vi "2P_AdapUprite_Linlin.vi"() -> ()   [LabVIEW 2015] (continued)
                                n1300 = local read "avpp"() -> (w4003:i32)
                                n1301 = call "tt_timeandsamples.vi"("bin"=w3997, "refreshtime"=w3991, "srateAODOtt"=w3994, "tot#ofsamples"=w3999) -> ("refreshrate"=w3995:dbl, "refreshbuffer"=w3996:i32, "timetracecycles"=w4001:i32)  [unwired: 5 in]
                                n1302 = local read "bin"() -> (w3998:dbl)
                                n1303 = call "2pparameters.vi"("command"="get") -> ("params out"=w4010:T12)  [unwired: 1 in]
                                n1304 = Bundle By Name(cluster=w4010, "Drawing Mode"=w3971, "measpoints"=w3999, "tt_cycles"=w4001, "refreshbuffer"=w3996, "refreshrate"=w3995, "Vx-ref"=w4002, "Vy-ref"=w4004, "srate"=w3993, "finite"=w4006, "cont"=w4005, "wavdet"=w4007, "avpp"=w4003, "srateAODO"=w4000, "bufferAI"=w3996, "bin"=w3998, "Angle Img"=w3978, "Vxminref"=w3977, "Vxmaxref"=w3976, "Vyminref"=w3975, "Vymaxref"=w3974, "Xpixels Img"=w3973, "Ypixels Img"=w3972, "Pel"=w3970, "Vz-reset"=0.0, "AIoverride"=w3968) -> (w4008:T12)
                                n1305 = Reciprocal(x=w3995) -> (1/x=w3992:dbl)
                                n1306 = local write "refreshtime"(w3992) -> ()
                                n1307 = call "2pparameters.vi"("Params in"=w4008, "command"="set") -> ()  [unwired: 1 out]
                                n1308 = local read "Voltage Clamp"() -> (w3985:bool)
                                n1309 = local read "Current Clamp"() -> (w3986:bool)
                                n1310 = local read "Vholding (mV)"() -> (w3980:sgl)
                                n1311 = local read "CC_ICgain"() -> (w3984:dbl)
                                n1312 = local read "OCgain"() -> (w3981:sgl)
                                n1313 = local read "holdon"() -> (w3979:bool)
                                n1314 = call "patchparameters.vi"("command"="get") -> ("Params out"=w3988:T16)  [unwired: 1 in]
                                n1315 = Bundle By Name(cluster=w3988, "VC"=w3985, "CC"=w3986, "CC_icg (pA/mv)"=w3984, "VC_icg (mV/mV)"=10.0, "OCG (mV/pA)"=w3981, "OVG (mV/mV)"=0.1, "Vhold (mV)"=w3980, "holdon"=w3979) -> (w3987:T16)
                                n1316 = call "patchparameters.vi"("Params in"=w3987, "command"="set") -> ()  [unwired: 1 out]
                              }
                              frame #4 {
                                # "calculating the waveform from the drawing"
                                n1317 = case shown="\"freeform contour\"" w4012 {
                                frame "Point" {
                                n1318 = call "2pparameters.vi"("command"="get") -> ("params out"=w4028:T12)  [unwired: 1 in]
                                n1319 = Unbundle By Name(w4028) -> ("Pel"=w4017:sgl, "Vx-min Img"=w4030:dbl, "VX-max Img"=w4029:dbl, "Vy-min Img"=w4032:dbl, "Vy-max Img"=w4031:dbl, "Angle Img"=w4033:dbl, "Vx-ref"=w4026:dbl, "Vy-ref"=w4025:dbl)
                                n1320 = script code="Xic=(ximax+ximin)./2;\nYic=(yimax+yimin)./2;\nx=x-Xic;\ny=y-Yic;\nxout=x.*cos(pi/180.*phi)+y.*sin(pi./180.*phi)+Xic;\nyout=-x.*sin(pi./180.*phi)+y.*cos(pi./180.*phi)+Yic;"("ximax"=w4029, "ximin"=w4030, "yimax"=w4031, "yimin"=w4032, "phi"=w4033, "x"=w4026, "y"=w4025) -> ("xout"=w4019:dbl, "yout"=w4018:dbl)  [unwired: 1 in, 1 out]
                                n1321 = call "2pparameters.vi"("command"="get") -> ("params out"=w4021:T12)  [unwired: 1 in]
                                n1322 = Bundle By Name(cluster=w4021, "P"=0.0) -> (w4024:T12)
                                n1323 = Initialize Array(w4018, w4017) -> (w4015:dbl[])
                                n1324 = Initialize Array(w4019, w4017) -> (w4014:dbl[])
                                n1325 = call "2pparameters.vi"("Params in"=w4024, "command"="set") -> ()  [unwired: 1 out]
                                n1326 = call "X-array-databuffer.vi"("array in"=w4014, "command"=enum16{"get", "set", "clear", "append"}."set") -> ()  [unwired: 2 in, 2 out]
                                n1327 = call "Y-array-databuffer.vi"("array in"=w4015, "command"=enum16{"get", "set", "clear", "append"}."set") -> ()  [unwired: 2 in, 2 out]
                                }
                                frame "Resonant Ellipse", Default {
                                n1328 = call "2pparameters.vi"("command"="get") -> ("params out"=w4048:T12)  [unwired: 1 in]
                                n1329 = Unbundle By Name(w4048) -> ("srateAODO"=w4049:sgl, "Angle Img"=w4050:dbl, "Angle draw"=w4051:dbl, "Vxmaxref"=w4052:dbl, "Vxminref"=w4053:dbl, "Xpixels Img"=w4054:i32, "Ypixels Img"=w4055:i32, "Vymaxref"=w4056:dbl, "Vyminref"=w4057:dbl, "Drawing Mode"=w4058:u16, "Pel"=w4059:sgl)
                                n1330 = Add(x=w4050, y=w4051) -> (x+y=w4034:dbl)
                                n1331 = call "ROI-databuffer.vi"("command"=enum16{"get", "set", "clear", "append"}."get") -> ("array out"=w4042:cluster{"x":sgl, "y":sgl}[])  [unwired: 4 in]
                                n1332 = call "ScanningWaveform_v4.vi"("Vy-min"=w4057, "Vy-max"=w4056, "yPixels/tPixels"=w4055, "xPixels/rPixels"=w4054, "Vx-min"=w4053, "Vx-max"=w4052, "Drawing Mode"=w4058, "Angle"=w4034, "AOrate"=w4049, "Points"=w4042, "points in ellipse"=w4059) -> ("numPixels"=w4035:dbl, "Y-WaveArray"=w4036:dbl[], "P"=w4041:dbl, "X-WaveArray"=w4037:dbl[])  [unwired: 5 in]
                                n1333 = call "Y-array-databuffer.vi"("array in"=w4036, "command"=enum16{"get", "set", "clear", "append"}."set") -> ()  [unwired: 2 in, 2 out]
                                n1334 = call "X-array-databuffer.vi"("array in"=w4037, "command"=enum16{"get", "set", "clear", "append"}."set") -> ()  [unwired: 2 in, 2 out]
                                n1335 = call "2pparameters.vi"("command"="get") -> ("params out"=w4046:T12)  [unwired: 1 in]
                                n1336 = Bundle By Name(cluster=w4046, "P"=w4041, "sAOxy"=w4035, "Pel"=w4035) -> (w4038:T12)
                                n1337 = call "2pparameters.vi"("Params in"=w4038, "command"="set") -> ()  [unwired: 1 out]
                                }
                                frame "freeform contour" {
                                n1338 = disable-structure shown="Enabled" {
                                frame Disabled {
                                # "Started writing this because old one was crashing....\nI think I found the source of the crash and was able to fix old one\n-Simon"
                                n1339 = call "2pparameters.vi"("command"="get") -> ("params out"=w4073:T12)  [unwired: 1 in]
                                n1340 = Unbundle By Name(w4073) -> ("Pel"=w4062:sgl)  [unwired: 10 out]
                                n1341 = call "ROI-databuffer.vi"("command"=enum16{"get", "set", "clear", "append"}."get") -> ("array out"=w4063:cluster{"x":sgl, "y":sgl}[])  [unwired: 4 in]
                                n1342 = call "Contour_ToVolts.vi"("N Contour Points"=w4062, "Array In"=w4063) -> ("Y Array Out"=w4060:dbl[], "X Array Out"=w4061:dbl[])  [unwired: 8 in]
                                n1343 = call "2pparameters.vi"("command"="get") -> ("params out"=w4071:T12)  [unwired: 1 in]
                                n1344 = Bundle By Name(cluster=w4071, "P"=0.0, "sAOxy"=w4062, "Pel"=w4062) -> (w4065:T12)
                                n1345 = call "Y-array-databuffer.vi"("array in"=w4060, "command"=enum16{"get", "set", "clear", "append"}."set") -> ()  [unwired: 2 in, 2 out]
                                n1346 = call "X-array-databuffer.vi"("array in"=w4061, "command"=enum16{"get", "set", "clear", "append"}."set") -> ()  [unwired: 2 in, 2 out]
                                n1347 = call "2pparameters.vi"("Params in"=w4065, "command"="set") -> ()  [unwired: 1 out]
                                }
                                frame Enabled {
                                n1348 = call "2pparameters.vi"("command"="get") -> ("params out"=w4088:T12)  [unwired: 1 in]
                                n1349 = Unbundle By Name(w4088) -> ("srateAODO"=w4089:sgl, "Angle Img"=w4090:dbl, "Angle draw"=w4091:dbl, "Vxmaxref"=w4092:dbl, "Vxminref"=w4093:dbl, "Xpixels Img"=w4094:i32, "Ypixels Img"=w4095:i32, "Vymaxref"=w4096:dbl, "Vyminref"=w4097:dbl, "Drawing Mode"=w4098:u16, "Pel"=w4099:sgl)
                                n1350 = Add(x=w4090, y=w4091) -> (x+y=w4074:dbl)
                                n1351 = call "ROI-databuffer.vi"("command"=enum16{"get", "set", "clear", "append"}."get") -> ("array out"=w4082:cluster{"x":sgl, "y":sgl}[])  [unwired: 4 in]
                                n1352 = call "ScanningWaveform_v4.vi"("Vy-min"=w4097, "Vy-max"=w4096, "yPixels/tPixels"=w4095, "xPixels/rPixels"=w4094, "Vx-min"=w4093, "Vx-max"=w4092, "Drawing Mode"=w4098, "Angle"=w4074, "AOrate"=w4089, "Points"=w4082, "points in ellipse"=w4099) -> ("numPixels"=w4075:dbl, "Y-WaveArray"=w4076:dbl[], "P"=w4081:dbl, "X-WaveArray"=w4077:dbl[])  [unwired: 5 in]
                                n1353 = call "Y-array-databuffer.vi"("array in"=w4076, "command"=enum16{"get", "set", "clear", "append"}."set") -> ()  [unwired: 2 in, 2 out]
                                n1354 = call "X-array-databuffer.vi"("array in"=w4077, "command"=enum16{"get", "set", "clear", "append"}."set") -> ()  [unwired: 2 in, 2 out]
                                n1355 = call "2pparameters.vi"("command"="get") -> ("params out"=w4086:T12)  [unwired: 1 in]
                                n1356 = Bundle By Name(cluster=w4086, "P"=w4081, "sAOxy"=w4075, "Pel"=w4075) -> (w4078:T12)
                                n1357 = call "2pparameters.vi"("Params in"=w4078, "command"="set") -> ()  [unwired: 1 out]
                                }
                                }
                                }
                                }
                              }
                              frame #5 {
                                # "set starting position"
                                n1358 = call "X-array-databuffer.vi"("command"=enum16{"get", "set", "clear", "append"}."get") -> ("array out"=w4102:dbl[])  [unwired: 3 in, 1 out]
                                n1359 = call "Y-array-databuffer.vi"("command"=enum16{"get", "set", "clear", "append"}."get") -> ("array out"=w4105:dbl[])  [unwired: 3 in, 1 out]
                                n1360 = Index Array(array=w4102, index=0) -> (element=w4101:dbl)
                                n1361 = Index Array(array=w4105, index=0) -> (element=w4100:dbl)
                                n1362 = call "setposition.vi"("Vy"=w4100, "Vx"=w4101) -> ()  [unwired: 1 in]
                              }
                              frame #6 {
                                # "rem2Ps"
                                # "A2Ps"
                                # "Al"
                                # "Rl"
                                # "Here it is writing the contour to a waveform that will be given to the AO (and also DO)"
                                n1363 = stacked-sequence {
                                seq-local: [w4126 _ _ _ _ _ _ _ _ _ _] -> [_ w4246 _ w4307 _ w4393 _ _ _ _ _]
                                seq-local: [w4127 _ _ _ _ _ _ _ _ _ _] -> [_ w4247 w4257 _ w4362 _ _ _ _ _ _]
                                seq-local: [_ _ w4256 _ _ _ _ _ _ _ _] -> [_ _ _ _ w4356 _ _ _ _ _ _]
                                seq-local: [_ _ _ w4306 _ _ _ _ _ _ _] -> [_ _ _ _ _ w4392 _ _ _ _ _]
                                seq-local: [w4123 _ _ _ _ _ _ _ _ _ _] -> [_ w4243 _ _ _ _ _ _ w4602 w4670 _]
                                seq-local: [w4122 _ _ _ _ _ _ _ _ _ _] -> [_ w4242 _ _ _ _ _ _ w4603 w4671 _]
                                seq-local: [w4129 _ _ _ _ _ _ _ _ _ _] -> [_ _ _ _ _ _ w4427 _ w4601 w4669 _]
                                seq-local: [w4125 _ _ _ _ _ _ _ _ _ _] -> [_ w4241 _ _ _ _ w4429 w4510 _ _ _]
                                seq-local: [w4124 _ _ _ _ _ _ _ _ _ _] -> [_ w4240 _ _ _ _ w4428 w4509 _ _ _]
                                seq-local: [w4128 _ _ _ _ _ _ _ _ _ _] -> [_ _ _ _ _ _ w4430 w4506 _ _ _]
                                tunnel: [_ _ w4255 _ _ _ _ _ _ _ _] -> w4120
                                tunnel: [_ _ w4254 _ _ _ _ _ _ _ _] -> w4121
                                tunnel: [w4127 _ _ _ _ _ _ _ _ _ _] -> w4119
                                tunnel: [w4126 _ _ _ _ _ _ _ _ _ _] -> w4116
                                tunnel: [_ _ _ w4305 _ _ _ _ _ _ _] -> w4117
                                tunnel: [_ _ _ w4304 _ _ _ _ _ _ _] -> w4118
                                tunnel: [w4125 _ _ _ _ _ _ _ _ _ _] -> w4111
                                tunnel: [w4124 _ _ _ _ _ _ _ _ _ _] -> w4110
                                tunnel: [_ _ _ _ _ _ w4431 _ _ _ _] -> w4109
                                tunnel: [_ _ _ _ _ _ _ w4507 _ _ _] -> w4108
                                tunnel: [w4123 _ _ _ _ _ _ _ _ _ _] -> w4112
                                tunnel: [w4122 _ _ _ _ _ _ _ _ _ _] -> w4113
                                tunnel: [_ _ _ _ _ _ _ _ w4600 _ _] -> w4114
                                tunnel: [_ _ _ _ _ _ _ _ _ w4668 _] -> w4115
                                frame #0 {
                                # "for a next version, give ome thought to\nthe possibilit of intermittently updating the\nwaveforms. it will have to be a calculation\nbased on speed of CPU and program on the one hand\nand length of measurement on the other. but then it should be possible, in principle, to \nupdate the waveform on the fly and that way cut up a longer measurement in smaller parts."
                                n1364 = stacked-sequence {
                                tunnel: [w4132 _ _ _] -> w4127
                                tunnel: [_ w4144 _ _] -> w4126
                                tunnel: [_ _ _ w4207] -> w4122
                                tunnel: [_ _ _ w4206] -> w4123
                                tunnel: [_ _ _ w4205] -> w4129
                                tunnel: [_ _ w4155 _] -> w4125
                                tunnel: [_ _ w4154 _] -> w4124
                                tunnel: [_ _ w4156 _] -> w4128
                                frame #0 {
                                n1365 = call "configuration_2P_Linlin.vi"("command"="get") -> ("config out"=w4130:T14)  [unwired: 2 in, 1 out]
                                n1366 = call "2pparameters.vi"("command"="get") -> ("params out"=w4136:T12)  [unwired: 1 in]
                                n1367 = Unbundle By Name(w4130) -> ("Voltage to Xgalvo"=w4133:i32)
                                n1368 = in-place {
                                in-place-border: w4133 -> [w4141]
                                in-place-border: [w4138] -> w4132
                                n1369 = in-place-cluster #23(w4136) -> ("aAO"=w4140:u32[])
                                n1370 = call "add channel to active arrayv2.vi"("line array in"=w4140, "line to add"=w4141) -> ("line array out"=w4139:u32[], "addition"=w4138:bool)  [unwired: 1 out]
                                n1371 = in-place-cluster #23("aAO"=w4139) -> (w4134:T12)
                                }
                                n1372 = call "2pparameters.vi"("Params in"=w4134, "command"="set") -> ()  [unwired: 1 out]
                                }
                                frame #1 {
                                n1373 = call "configuration_2P_Linlin.vi"("command"="get") -> ("config out"=w4142:T14)  [unwired: 2 in, 1 out]
                                n1374 = Unbundle By Name(w4142) -> ("Voltage to Ygalvo"=w4145:i32)
                                n1375 = call "2pparameters.vi"("command"="get") -> ("params out"=w4148:T12)  [unwired: 1 in]
                                n1376 = in-place {
                                in-place-border: w4145 -> [w4153]
                                in-place-border: [w4150] -> w4144
                                n1377 = in-place-cluster #24(w4148) -> ("aAO"=w4152:u32[])
                                n1378 = call "add channel to active arrayv2.vi"("line array in"=w4152, "line to add"=w4153) -> ("line array out"=w4151:u32[], "addition"=w4150:bool)  [unwired: 1 out]
                                n1379 = in-place-cluster #24("aAO"=w4151) -> (w4146:T12)
                                }
                                n1380 = call "2pparameters.vi"("Params in"=w4146, "command"="set") -> ()  [unwired: 1 out]
                                }
                                frame #2 {
                                n1381 = call "2pparameters.vi"("command"="get") -> ("params out"=w4159:T12)  [unwired: 1 in]
                                n1382 = Unbundle By Name(w4159) -> ("autoshutter"=w4158:bool, "wavdet"=w4157:bool)
                                n1383 = case shown="True" w4158 {
                                tunnel: [w4164 w4187] -> w4155
                                tunnel: [w4163 FALSE ("removal")] -> w4154
                                tunnel: [w4162 w4186] -> w4156
                                tunnel: w4157 -> [w4161 _]
                                frame False {
                                n1384 = case shown="False" w4161 {
                                tunnel: [FALSE ("addition") FALSE ("addition")] -> w4164
                                tunnel: [w4168 FALSE ("removal")] -> w4163
                                tunnel: [w4167 _] -> w4162
                                frame False {
                                n1385 = call "2pparameters.vi"("command"="get") -> ("params out"=w4166:T12)  [unwired: 1 in]
                                n1386 = Unbundle By Name(w4166) -> ("aAS"=w4165:u32[])
                                n1387 = in-place {
                                in-place-border: [w4173] -> w4168
                                in-place-border: [w4176] -> w4167
                                in-place-border: w4165 -> [w4175]
                                n1388 = in-place-cluster #25(w4166) -> ("aDO"=w4178:u32[])
                                n1389 = for {
                                tunnel: [w4181] -> w4174 mode=indexing
                                tunnel: [w4180] -> w4176 mode=indexing
                                shift-right: [w4182] -> w4177
                                shift-left: w4178 -> [w4183]
                                tunnel: w4175 -> [w4179] mode=indexing
                                n1390 = call "remove channel from active arrayv2.vi"("line array in"=w4183, "line to remove"=w4179) -> ("line array out"=w4182:u32[], "removal"=w4181:bool, "index"=w4180:i32)
                                }
                                n1391 = Or Array Elements(Boolean array=w4174) -> (logical OR=w4173:bool)
                                n1392 = in-place-cluster #25("aDO"=w4177) -> (w4169:T12)
                                }
                                n1393 = call "2pparameters.vi"("Params in"=w4169, "command"="set") -> ()  [unwired: 1 out]
                                }
                                frame True {
                                }
                                }
                                }
                                frame True {
                                n1394 = call "2pparameters.vi"("command"="get") -> ("params out"=w4189:T12)  [unwired: 1 in]
                                n1395 = Unbundle By Name(w4189) -> ("aAS"=w4188:u32[])
                                n1396 = in-place {
                                in-place-border: w4188 -> [w4199]
                                in-place-border: [w4195] -> w4187
                                in-place-border: [w4194] -> w4186
                                n1397 = in-place-cluster #26(w4189) -> ("aDO"=w4198:u32[])
                                n1398 = for {
                                tunnel: w4199 -> [w4204] mode=indexing
                                shift-right: [w4202] -> w4197
                                shift-left: w4198 -> [w4203]
                                tunnel: [w4201] -> w4196 mode=indexing
                                tunnel: [w4200] -> w4194 mode=indexing
                                n1399 = call "add channel to active arrayv2.vi"("line array in"=w4203, "line to add"=w4204) -> ("line array out"=w4202:u32[], "addition"=w4201:bool, "index"=w4200:i32)
                                }
                                n1400 = Or Array Elements(Boolean array=w4196) -> (logical OR=w4195:bool)
                                n1401 = in-place-cluster #26("aDO"=w4197) -> (w4191:T12)
                                }
                                n1402 = call "2pparameters.vi"("Params in"=w4191, "command"="set") -> ()  [unwired: 1 out]
                                }
                                }
                                }
                                frame #3 {
                                n1403 = local read "Measurement"() -> (w4208:T4)
                                n1404 = To Unsigned Long Integer(number=w4208) -> (unsigned 32bit integer=w4209:u32)
                                n1405 = case shown="5..7" w4209 {
                                tunnel: [FALSE ("addition") w4229] -> w4207
                                tunnel: [w4214 FALSE ("removal")] -> w4206
                                tunnel: [w4212 w4227] -> w4205
                                frame 0..4, Default {
                                n1406 = call "configuration_2P_Linlin.vi"("command"="get") -> ("config out"=w4210:T14)  [unwired: 2 in, 1 out]
                                n1407 = Unbundle By Name(w4210) -> ("LT timestamp"=w4217:u32)
                                n1408 = call "2pparameters.vi"("command"="get") -> ("params out"=w4218:T12)  [unwired: 1 in]
                                n1409 = in-place {
                                in-place-border: w4217 -> [w4224]
                                in-place-border: [w4221] -> w4214
                                in-place-border: [w4220] -> w4212
                                n1410 = in-place-cluster #27(w4218) -> ("aDO"=w4223:u32[])
                                n1411 = call "remove channel from active arrayv2.vi"("line array in"=w4223, "line to remove"=w4224) -> ("line array out"=w4222:u32[], "removal"=w4221:bool, "index"=w4220:i32)
                                n1412 = in-place-cluster #27("aDO"=w4222) -> (w4215:T12)
                                }
                                n1413 = call "2pparameters.vi"("Params in"=w4215, "command"="set") -> ()  [unwired: 1 out]
                                }
                                frame 5..7 {
                                n1414 = call "configuration_2P_Linlin.vi"("command"="get") -> ("config out"=w4225:T14)  [unwired: 2 in, 1 out]
                                n1415 = Unbundle By Name(w4225) -> ("LT timestamp"=w4232:u32)
                                n1416 = call "2pparameters.vi"("command"="get") -> ("params out"=w4233:T12)  [unwired: 1 in]
                                n1417 = in-place {
                                in-place-border: w4232 -> [w4239]
                                in-place-border: [w4236] -> w4229
                                in-place-border: [w4235] -> w4227
                                n1418 = in-place-cluster #28(w4233) -> ("aDO"=w4238:u32[])
                                n1419 = call "add channel to active arrayv2.vi"("line array in"=w4238, "line to add"=w4239) -> ("line array out"=w4237:u32[], "addition"=w4236:bool, "index"=w4235:i32)
                                n1420 = in-place-cluster #28("aDO"=w4237) -> (w4230:T12)
                                }
                                n1421 = call "2pparameters.vi"("Params in"=w4230, "command"="set") -> ()  [unwired: 1 out]
                                }
                                }
                                }
                                }
                                }
                                frame #1 {
                                n1422 = Or(x=w4246, y=w4247) -> (x .or. y?=w4245:bool)
                                n1423 = case shown="True" w4245 {
                                frame False {
                                }
                                frame True {
                                # "update GUI"
                                n1424 = call "Used AO lines.vi"() -> ("used AO names"=w4251:string[], "used AO lines"=w4253:tag[])  [unwired: 2 in]
                                n1425 = control-ref of="Analog Lines Plot"() -> (w4252:refnum<vi>)
                                n1426 = local write "Analog Used Lines"(w4253) -> ()
                                n1427 = local write "Analog Used Names"(w4251) -> ()
                                n1428 = call "prepAOWaveplot.vi"("WaveformGraph in"=w4252, "Analog Used Names"=w4251) -> ()  [unwired: 1 in]
                                }
                                }
                                n1429 = Compound Arithmetic op=OR(w4243, w4242, w4241, w4240) -> (w4244:bool)
                                n1430 = case shown="True" w4244 {
                                frame False {
                                }
                                frame True {
                                n1431 = control-ref of="Digital Lines Plot"() -> (w4248:refnum<vi>)
                                n1432 = call "Used DO lines.vi"() -> ("used DO names"=w4249:string[], "used DO lines"=w4250:tag[])  [unwired: 2 in]
                                n1433 = local write "Digital Used Lines"(w4250) -> ()
                                n1434 = local write "Digital Used Names"(w4249) -> ()
                                n1435 = call "prepDOWaveplot.vi"("DigitalGraph in"=w4248, "used DO names"=w4249) -> ()  [unwired: 1 in]
                                }
                                }
                                }
                                frame #2 {
                                n1436 = case shown="True" w4257 {
                                tunnel: [w4260 w4288] -> w4256
                                tunnel: [w4259 w4286] -> w4255
                                tunnel: [w4258 _] -> w4254
                                frame False {
                                n1437 = stacked-sequence {
                                seq-local: [w4264 _] -> [_ w4277]
                                tunnel: [w4264 _] -> w4260
                                tunnel: [w4267 _] -> w4259
                                tunnel: [w4263 _] -> w4258
                                frame #0 {
                                n1438 = call "configuration_2P_Linlin.vi"("command"="get") -> ("config out"=w4261:T14)  [unwired: 2 in, 1 out]
                                n1439 = call "waveformparamsv2.vi"("command"="get") -> ("Params out"=w4269:T17)  [unwired: 4 in, 2 out]
                                n1440 = Unbundle By Name(w4261) -> ("Voltage to Xgalvo"=w4274:i32)
                                n1441 = call "2pparameters.vi"("command"="get") -> ("params out"=w4272:T12)  [unwired: 1 in]
                                n1442 = Unbundle By Name(w4269) -> ("AO parameters"=w4268:T18)
                                n1443 = Unbundle By Name(w4272) -> ("aAO"=w4273:u32[])
                                n1444 = call "waveformsAObuffer.vi"("command"="get") -> ("AO wf out"=w4265:waveform(dbl)[])  [unwired: 1 in]
                                n1445 = Search 1D Array(1D array=w4273, element=w4274) -> (index of element=w4264:i32)  [unwired: 1 in]
                                n1446 = Index Array(array=w4265, index=w4264) -> (element=w4263:waveform(dbl))
                                n1447 = Index Array(array=w4268, index=w4264) -> (element=w4267:T19)
                                }
                                frame #1 {
                                w4278 = 0.0 ("Step size (V)")
                                n1448 = local read "Meastab"() -> (w4276:enum32{"X-Y Image", "Linescan", "Timetrace"})
                                n1449 = case shown="\"X-Y Image\", Default" w4276 {
                                tunnel: [w4280 w4281] -> w4275
                                frame "X-Y Image", Default {
                                n1450 = local read "Sampling rate"() -> (w4280:dbl)
                                }
                                frame "Timetrace" {
                                n1451 = local read "srateAODOtt"() -> (w4281:dbl)
                                }
                                }
                                n1452 = call "replace AO XYwfparam.vi"("Baseline (V)"=w4278, "Start amplitude (V)"=w4278, "Cycles"=w4278, "Repeats"=w4278, "index of AO wave"=w4277, "Step size (V)"=w4278, "DC (%)"=w4278, "Sampling frequency (Hz)"=w4275, "Period (ms)"=w4278, "Cycle length (s)"=w4278, "Pulses"=w4278, "padding value"=w4278, "Matlab wave name"=path "xwave") -> ()  [unwired: 3 in]
                                }
                                }
                                }
                                frame True {
                                w4287 = 0.0 ("Repeats")
                                n1453 = local read "Meastab"() -> (w4285:enum32{"X-Y Image", "Linescan", "Timetrace"})
                                n1454 = case shown="\"Timetrace\"" w4285 {
                                tunnel: [w4302 w4303] -> w4284
                                frame "X-Y Image", Default {
                                n1455 = local read "Sampling rate"() -> (w4302:dbl)
                                }
                                frame "Timetrace" {
                                n1456 = local read "srateAODOtt"() -> (w4303:dbl)
                                }
                                }
                                n1457 = call "2pparameters.vi"("command"="get") -> ("params out"=w4290:T12)  [unwired: 1 in]
                                n1458 = call "waveformparamsv2.vi"("command"="get") -> ("Params out"=w4299:T17)  [unwired: 4 in, 2 out]
                                n1459 = call "configuration_2P_Linlin.vi"("command"="get") -> ("config out"=w4283:T14)  [unwired: 2 in, 1 out]
                                n1460 = Unbundle By Name(w4283) -> ("Voltage to Xgalvo"=w4292:i32)
                                n1461 = Unbundle By Name(w4299) -> ("AO parameters"=w4296:T18)
                                n1462 = Unbundle By Name(w4290) -> ("aAO"=w4291:u32[])
                                n1463 = Search 1D Array(1D array=w4291, element=w4292) -> (index of element=w4288:i32)  [unwired: 1 in]
                                n1464 = Index Array(array=w4296, index=0) -> (element=w4297:T19)
                                n1465 = Bundle By Name(cluster=w4297, "AOtab"=-1.0 ("Repeats"), "Repeats"=w4287, "Cycles"=w4287, "Start amplitude (V)"=w4287, "Baseline (V)"=w4287, "Step size (V)"=w4287, "DC (%)"=w4287, "Sampling frequency (Hz)"=w4284, "Period (ms)"=w4287, "Offset (V)"=w4287, "Amplitude (V)"=w4287, "Frequency"=w4287, "Tri Repeats"=w4287, "phase shift (ms)"=w4287, "Pulses"=w4287, "Matlab wave file"=path "xwave", "padding value"=w4287) -> (w4286:T19)
                                n1466 = Build Array(w4286) -> (w4294:T18)
                                n1467 = call "waveformparamsv2.vi"("command"="add AO", "add AO"=w4294) -> ()  [unwired: 3 in, 3 out]
                                }
                                }
                                }
                                frame #3 {
                                n1468 = case shown="True" w4307 {
                                tunnel: [w4310 w4338] -> w4306
                                tunnel: [w4309 w4336] -> w4305
                                tunnel: [w4308 _] -> w4304
                                frame False {
                                n1469 = stacked-sequence {
                                seq-local: [w4314 _] -> [_ w4327]
                                tunnel: [w4314 _] -> w4310
                                tunnel: [w4317 _] -> w4309
                                tunnel: [w4313 _] -> w4308
                                frame #0 {
                                n1470 = call "configuration_2P_Linlin.vi"("command"="get") -> ("config out"=w4311:T14)  [unwired: 2 in, 1 out]
                                n1471 = call "waveformparamsv2.vi"("command"="get") -> ("Params out"=w4319:T17)  [unwired: 4 in, 2 out]
                                n1472 = Unbundle By Name(w4311) -> ("Voltage to Ygalvo"=w4324:i32)
                                n1473 = call "2pparameters.vi"("command"="get") -> ("params out"=w4322:T12)  [unwired: 1 in]
                                n1474 = Unbundle By Name(w4319) -> ("AO parameters"=w4318:T18)
                                n1475 = Unbundle By Name(w4322) -> ("aAO"=w4323:u32[])
                                n1476 = call "waveformsAObuffer.vi"("command"="get") -> ("AO wf out"=w4315:waveform(dbl)[])  [unwired: 1 in]
                                n1477 = Search 1D Array(1D array=w4323, element=w4324) -> (index of element=w4314:i32)  [unwired: 1 in]
                                n1478 = Index Array(array=w4315, index=w4314) -> (element=w4313:waveform(dbl))
                                n1479 = Index Array(array=w4318, index=w4314) -> (element=w4317:T19)
                                }
                                frame #1 {
                                w4328 = 0.0 ("Step size (V)")
                                n1480 = local read "Meastab"() -> (w4326:enum32{"X-Y Image", "Linescan", "Timetrace"})
                                n1481 = case shown="\"X-Y Image\", Default" w4326 {
                                tunnel: [w4330 w4331] -> w4325
                                frame "X-Y Image", Default {
                                n1482 = local read "Sampling rate"() -> (w4330:dbl)
                                }
                                frame "Timetrace" {
                                n1483 = local read "srateAODOtt"() -> (w4331:dbl)
                                }
                                }
                                n1484 = call "replace AO XYwfparam.vi"("Baseline (V)"=w4328, "Start amplitude (V)"=w4328, "Cycles"=w4328, "Repeats"=w4328, "index of AO wave"=w4327, "Step size (V)"=w4328, "DC (%)"=w4328, "Sampling frequency (Hz)"=w4325, "Period (ms)"=w4328, "Cycle length (s)"=w4328, "Pulses"=w4328, "padding value"=w4328, "Matlab wave name"=path "ywave") -> ()  [unwired: 3 in]
                                }
                                }
                                }
                                frame True {
                                w4337 = 0.0 ("Repeats")
                                n1485 = local read "Meastab"() -> (w4335:enum32{"X-Y Image", "Linescan", "Timetrace"})
                                n1486 = case shown="\"X-Y Image\", Default" w4335 {
                                tunnel: [w4352 w4353] -> w4334
                                frame "X-Y Image", Default {
                                n1487 = local read "Sampling rate"() -> (w4352:dbl)
                                }
                                frame "Timetrace" {
                                n1488 = local read "srateAODOtt"() -> (w4353:dbl)
                                }
                                }
                                n1489 = call "2pparameters.vi"("command"="get") -> ("params out"=w4340:T12)  [unwired: 1 in]
                                n1490 = call "waveformparamsv2.vi"("command"="get") -> ("Params out"=w4350:T17)  [unwired: 4 in, 2 out]
                                n1491 = call "configuration_2P_Linlin.vi"("command"="get") -> ("config out"=w4332:T14)  [unwired: 2 in, 1 out]
                                n1492 = Unbundle By Name(w4332) -> ("Voltage to Ygalvo"=w4342:i32)
                                n1493 = Unbundle By Name(w4350) -> ("AO parameters"=w4347:T18)
                                n1494 = Unbundle By Name(w4340) -> ("aAO"=w4341:u32[])
                                n1495 = Search 1D Array(1D array=w4341, element=w4342) -> (index of element=w4338:i32)  [unwired: 1 in]
                                n1496 = Index Array(array=w4347, index=0) -> (element=w4348:T19)
                                n1497 = Bundle By Name(cluster=w4348, "AOtab"=-1.0 ("Repeats"), "Repeats"=w4337, "Cycles"=w4337, "Start amplitude (V)"=w4337, "Baseline (V)"=w4337, "Step size (V)"=w4337, "DC (%)"=w4337, "Sampling frequency (Hz)"=w4334, "Period (ms)"=w4337, "Offset (V)"=w4337, "Amplitude (V)"=w4337, "Frequency"=w4337, "Tri Repeats"=w4337, "phase shift (ms)"=w4337, "Pulses"=w4337, "Matlab wave file"=path "ywave", "padding value"=w4337) -> (w4336:T19)
                                n1498 = Build Array(w4336) -> (w4345:T18)
                                n1499 = call "waveformparamsv2.vi"("command"="add AO", "add AO"=w4345) -> ()  [unwired: 3 in, 3 out]
                                }
                                }
                                }
                                frame #4 {
                                n1500 = call "2pparameters.vi"("command"="get") -> ("params out"=w4359:T12)  [unwired: 1 in]
                                n1501 = Unbundle By Name(w4359) -> ("wavdet"=w4358:bool, "Pel"=w4355:sgl, "refwfsize"=w4354:dbl, "srateAODO"=w4357:sgl)
                                n1502 = case shown="True" w4358 {
                                tunnel: [w4363 w4373] -> w4361
                                tunnel: w4357 -> [w4364 w4375]
                                tunnel: w4355 -> [_ w4371]
                                tunnel: w4354 -> [_ w4370]
                                frame False {
                                n1503 = call "X-array-databuffer.vi"("command"=enum16{"get", "set", "clear", "append"}."get") -> ("array out"=w4367:dbl[])  [unwired: 3 in, 1 out]
                                n1504 = Reciprocal(x=w4364) -> (1/x=w4365:sgl)
                                n1505 = Bundle By Name("Y"=w4367, "dt"=w4365) -> (w4363:waveform(dbl))  [unwired: 1 in]
                                }
                                frame True {
                                n1506 = To Double Precision Float(number=w4371) -> (double precision float=w4372:dbl)
                                n1507 = Divide(x=w4370, y=w4372) -> (x/y=w4369:dbl)
                                n1508 = Round Toward +Infinity(x=w4369) -> (ceil(x): smallest int >= x=w4368:dbl)
                                n1509 = call "X-array-databuffer.vi"("command"=enum16{"get", "set", "clear", "append"}."get") -> ("array out"=w4377:dbl[])  [unwired: 3 in, 1 out]
                                n1510 = Reciprocal(x=w4375) -> (1/x=w4376:sgl)
                                n1511 = for {
                                N: w4368 -> [_]
                                tunnel: w4377 -> [w4379]
                                tunnel: [w4379] -> w4374 mode=concatenating
                                }
                                n1512 = Bundle By Name("Y"=w4374, "dt"=w4376) -> (w4373:waveform(dbl))  [unwired: 1 in]
                                }
                                }
                                n1513 = case shown="True" w4362 {
                                tunnel: w4361 -> [w4381 w4387]
                                tunnel: w4356 -> [w4382 _]
                                frame False {
                                n1514 = call "waveformsAObuffer.vi"("command"="get") -> ("AO wf out"=w4385:waveform(dbl)[])  [unwired: 1 in]
                                n1515 = property on="refwf" class="Ring (strict)" props=["RingText", "Text"]() -> ()  [unwired: 2 in, 3 out]
                                n1516 = Replace Array Subset(array=w4385, new element=w4381, index=w4382) -> (w4380:waveform(dbl)[])
                                n1517 = call "waveformsAObuffer.vi"("AO wf in"=w4380, "command"="set") -> ()  [unwired: 1 out]
                                }
                                frame True {
                                n1518 = call "waveformsAObuffer.vi"("command"="get") -> ("AO wf out"=w4389:waveform(dbl)[])  [unwired: 1 in]
                                n1519 = Build Array (concatenate)(w4389, w4387) -> (w4386:waveform(dbl)[])
                                n1520 = call "waveformsAObuffer.vi"("AO wf in"=w4386, "command"="set") -> ()  [unwired: 1 out]
                                }
                                }
                                }
                                frame #5 {
                                n1521 = call "2pparameters.vi"("command"="get") -> ("params out"=w4401:T12)  [unwired: 1 in]
                                n1522 = Unbundle By Name(w4401) -> ("wavdet"=w4400:bool, "Pel"=w4398:sgl, "refwfsize"=w4399:dbl, "srateAODO"=w4394:sgl)
                                n1523 = To Double Precision Float(number=w4398) -> (double precision float=w4397:dbl)
                                n1524 = Divide(x=w4399, y=w4397) -> (x/y=w4396:dbl)
                                n1525 = Round Toward +Infinity(x=w4396) -> (ceil(x): smallest int >= x=w4395:dbl)
                                n1526 = case shown="False" w4400 {
                                tunnel: [w4405 w4411] -> w4391
                                tunnel: w4395 -> [_ w4408]
                                tunnel: w4394 -> [w4406 w4413]
                                frame False {
                                n1527 = call "Y-array-databuffer.vi"("command"=enum16{"get", "set", "clear", "append"}."get") -> ("array out"=w4403:dbl[])  [unwired: 3 in, 1 out]
                                n1528 = Reciprocal(x=w4406) -> (1/x=w4407:sgl)
                                n1529 = Bundle By Name("Y"=w4403, "dt"=w4407) -> (w4405:waveform(dbl))  [unwired: 1 in]
                                }
                                frame True {
                                n1530 = call "Y-array-databuffer.vi"("command"=enum16{"get", "set", "clear", "append"}."get") -> ("array out"=w4409:dbl[])  [unwired: 3 in, 1 out]
                                n1531 = Reciprocal(x=w4413) -> (1/x=w4414:sgl)
                                n1532 = for {
                                N: w4408 -> [_]
                                tunnel: w4409 -> [w4415]
                                tunnel: [w4415] -> w4412 mode=concatenating
                                }
                                n1533 = Bundle By Name("Y"=w4412, "dt"=w4414) -> (w4411:waveform(dbl))  [unwired: 1 in]
                                }
                                }
                                n1534 = case shown="False" w4393 {
                                tunnel: w4391 -> [w4418 w4423]
                                tunnel: w4392 -> [w4419 _]
                                frame False {
                                n1535 = call "waveformsAObuffer.vi"("command"="get") -> ("AO wf out"=w4421:waveform(dbl)[])  [unwired: 1 in]
                                n1536 = Replace Array Subset(array=w4421, new element=w4418, index=w4419) -> (w4416:waveform(dbl)[])
                                n1537 = call "waveformsAObuffer.vi"("AO wf in"=w4416, "command"="set") -> ()  [unwired: 1 out]
                                }
                                frame True {
                                n1538 = call "waveformsAObuffer.vi"("command"="get") -> ("AO wf out"=w4425:waveform(dbl)[])  [unwired: 1 in]
                                n1539 = Build Array (concatenate)(w4425, w4423) -> (w4422:waveform(dbl)[])
                                n1540 = call "waveformsAObuffer.vi"("AO wf in"=w4422, "command"="set") -> ()  [unwired: 1 out]
                                }
                                }
                                }
                                frame #6 {
                                n1541 = Build Array(w4429, w4428) -> (w4433:bool[])
                                n1542 = Boolean Array To Number(Boolean array=w4433) -> (number=w4432:u32)
                                n1543 = case shown="2" w4432 {
                                tunnel: w4430 -> [w4437 w4458 _ w4476]
                                tunnel: [_ w4457 _ w4474] -> w4431
                                tunnel: w4427 -> [_ _ _ _]
                                frame 1 {
                                w4447 = 0.0 ("DOtab")
                                # "This is not correctly handling the digital channel out with multichannel\nautoshutter. It should be a for loop, and add a channel with the appropriate\nname for each autoshutter channel"
                                # "remove True; add False"
                                n1544 = call "2pparameters.vi"("command"="get") -> ("params out"=w4444:T12)  [unwired: 1 in]
                                n1545 = Unbundle By Name(w4444) -> ("srateAODO"=w4440:sgl, "Pel"=w4443:sgl)
                                n1546 = call "waveformparamsv2.vi"("command"="get") -> ("Params out"=w4453:T17)  [unwired: 4 in, 2 out]
                                n1547 = Unbundle By Name(w4453) -> ("DO parameters"=w4451:T20)
                                n1548 = To Double Precision Float(number=w4440) -> (double precision float=w4438:dbl)
                                n1549 = To Double Precision Float(number=w4440) -> (double precision float=w4439:dbl)
                                n1550 = To Double Precision Float(number=w4443) -> (double precision float=w4442:dbl)
                                n1551 = Divide(x=w4439, y=w4442) -> (x/y=w4441:dbl)
                                n1552 = Index Array(array=w4451, index=0) -> (element=w4450:T21)
                                n1553 = Bundle By Name(cluster=w4450, "Digital DC (%)"=100.0, "Digital phase"=w4447, "Digital Freq (Hz)"=w4441, "Sampling frequency (Hz)"=w4438, "Digital time offset (s)"=w4447, "padding value"=0.0, "matlab wave file"=path "2Pshutter", "DOtab"=0.0) -> (w4436:T21)
                                n1554 = Array Size(array=w4437) -> (size(s)=w4435:i32)
                                n1555 = Initialize Array(w4436, w4435) -> (w4434:T20)
                                n1556 = call "waveformparamsv2.vi"("command"="add DO", "add DO"=w4434) -> ()  [unwired: 3 in, 3 out]
                                }
                                frame 2 {
                                # "remove False; add True"
                                n1557 = call "waveformparamsv2.vi"("command"="get") -> ("Params out"=w4460:T17)  [unwired: 4 in, 2 out]
                                n1558 = in-place {
                                in-place-border: w4458 -> [w4464]
                                in-place-border: [w4463] -> w4457
                                n1559 = in-place-cluster #29(w4460) -> ("DO parameters"=w4466:T20)
                                n1560 = for {
                                tunnel: w4464 -> [w4470] mode=indexing
                                tunnel: [w4467] -> w4463 mode=indexing
                                shift-right: [w4471] -> w4465
                                shift-left: w4466 -> [w4472]
                                n1561 = Delete From Array(array=w4472, length=1, index=w4470) -> (deleted portion=w4469:T20, array with subset deleted=w4471:T20)
                                n1562 = Index Array(array=w4469, index=0) -> (element=w4467:T21)
                                }
                                n1563 = in-place-cluster #29("DO parameters"=w4465) -> (w4459:T17)
                                }
                                n1564 = call "waveformparamsv2.vi"("command"="set", "Params in"=w4459) -> ()  [unwired: 3 in, 3 out]
                                }
                                frame 3, Default {
                                # "Remove True; Add True"
                                }
                                frame 0 {
                                # "remove False ; add False"
                                n1565 = call "2pparameters.vi"("command"="get") -> ("params out"=w4478:T12)  [unwired: 1 in]
                                n1566 = Unbundle By Name(w4478) -> ("autoshutter"=w4477:bool, "wavdet"=w4475:bool)
                                n1567 = case shown="True" w4477 {
                                tunnel: w4476 -> [_ w4482]
                                tunnel: w4475 -> [_ w4481]
                                tunnel: [_ w4480] -> w4474
                                frame False {
                                }
                                frame True {
                                n1568 = case shown="False" w4481 {
                                tunnel: w4482 -> [w4484 _]
                                tunnel: [w4483 _] -> w4480
                                frame False {
                                n1569 = stacked-sequence {
                                tunnel: w4484 -> [w4486 w4493]
                                tunnel: [w4485 _] -> w4483
                                frame #0 {
                                n1570 = call "waveformparamsv2.vi"("command"="get") -> ("Params out"=w4488:T17)  [unwired: 4 in, 2 out]
                                n1571 = Unbundle By Name(w4488) -> ("DO parameters"=w4487:T20)
                                n1572 = for {
                                tunnel: w4487 -> [w4492]
                                tunnel: w4486 -> [w4491] mode=indexing
                                tunnel: [w4490] -> w4485 mode=indexing
                                n1573 = Index Array(array=w4492, index=w4491) -> (element=w4490:T21)
                                }
                                }
                                frame #1 {
                                n1574 = for {
                                tunnel: w4493 -> [w4504] mode=indexing
                                w4503 = 0.0 ("padding value")
                                n1575 = call "2pparameters.vi"("command"="get") -> ("params out"=w4501:T12)  [unwired: 1 in]
                                n1576 = Unbundle By Name(w4501) -> ("srate"=w4498:sgl, "Pel"=w4500:sgl)
                                n1577 = To Double Precision Float(number=w4498) -> (double precision float=w4496:dbl)
                                n1578 = To Double Precision Float(number=w4498) -> (double precision float=w4497:dbl)
                                n1579 = To Double Precision Float(number=w4500) -> (double precision float=w4499:dbl)
                                n1580 = Divide(x=w4497, y=w4499) -> (x/y=w4495:dbl)
                                n1581 = call "replace DO wf param.vi"("Digital Freq (Hz)"=w4495, "Digital DC (%)"=100.0, "Digital phase"=w4503, "Sampling frequency (Hz)"=w4496, "Digital time offset (s)"=w4503, "index of DO wave"=w4504, "padding value"=w4503, "matlab wave file"=path "2Pshutter" ("matlab wave number")) -> ()  [unwired: 3 in]
                                }
                                }
                                }
                                }
                                frame True {
                                }
                                }
                                }
                                }
                                }
                                }
                                }
                                frame #7 {
                                n1582 = Build Array(w4510, w4509) -> (w4511:bool[])
                                n1583 = Boolean Array To Number(Boolean array=w4511) -> (number=w4508:u32)
                                n1584 = case shown="0" w4508 {
                                tunnel: w4506 -> [w4513 w4558 _ w4569]
                                tunnel: [_ w4559 _ w4567] -> w4507
                                frame 1 {
                                n1585 = call "2pparameters.vi"("command"="get") -> ("params out"=w4520:T12)  [unwired: 1 in]
                                n1586 = Unbundle By Name(w4520) -> ("wavdet"=w4521:bool, "Pel"=w4523:sgl, "refwfsize"=w4524:dbl, "srate"=w4522:sgl)
                                n1587 = call "waveformsDObuffer.vi"("command"="get") -> ("DO wf out"=w4516:digitalwaveform[])  [unwired: 1 in]
                                n1588 = case shown="False" w4521 {
                                tunnel: [w4532 w4542] -> w4518
                                tunnel: w4522 -> [w4537 w4553]
                                tunnel: w4523 -> [w4531 w4546]
                                tunnel: w4524 -> [_ w4550]
                                frame False {
                                w4535 = u16 0 items=["unsigned binary", "offset binary", "2's complement"] ("data format (offset binary)")
                                n1589 = Initialize Array(sgl 1.0, w4531) -> (w4528:sgl[])
                                n1590 = Reciprocal(x=w4537) -> (1/x=w4538:sgl)
                                n1591 = Bundle By Name("Y"=w4528, "dt"=w4538) -> (w4533:waveform(sgl))  [unwired: 1 in]
                                n1592 = call-poly <vilib>:"Analog to Digital.vi"("data format (offset binary)"=w4535, "compress digital (T)"=TRUE, "full-scale range (pk-pk)"=1.0, "resolution (16 bit)"=1, "analog waveform"=w4533) -> ("digital waveform"=w4532:digitalwaveform)  [unwired: 3 in, 3 out]
                                }
                                frame True {
                                w4545 = u16 0 items=["unsigned binary", "offset binary", "2's complement"] ("data format (offset binary)")
                                n1593 = To Double Precision Float(number=w4546) -> (double precision float=w4551:dbl)
                                n1594 = Initialize Array(sgl 1.0, w4546) -> (w4539:sgl[])
                                n1595 = Divide(x=w4550, y=w4551) -> (x/y=w4548:dbl)
                                n1596 = Round Toward +Infinity(x=w4548) -> (ceil(x): smallest int >= x=w4549:dbl)
                                n1597 = for {
                                N: w4549 -> [_]
                                tunnel: w4539 -> [w4555]
                                tunnel: [w4555] -> w4552 mode=concatenating
                                }
                                n1598 = Reciprocal(x=w4553) -> (1/x=w4554:sgl)
                                n1599 = Bundle By Name("Y"=w4552, "dt"=w4554) -> (w4543:waveform(sgl))  [unwired: 1 in]
                                n1600 = call-poly <vilib>:"Analog to Digital.vi"("data format (offset binary)"=w4545, "compress digital (T)"=TRUE, "full-scale range (pk-pk)"=1.0, "resolution (16 bit)"=1, "analog waveform"=w4543) -> ("digital waveform"=w4542:digitalwaveform)  [unwired: 3 in, 3 out]
                                }
                                }
                                n1601 = Array Size(array=w4513) -> (size(s)=w4512:i32)
                                n1602 = for {
                                N: w4512 -> [_]
                                tunnel: w4518 -> [w4527]
                                shift-right: [w4525] -> w4514
                                shift-left: w4516 -> [w4526]
                                n1603 = Build Array (concatenate)(w4526, w4527) -> (w4525:digitalwaveform[])
                                }
                                n1604 = call "waveformsDObuffer.vi"("DO wf in"=w4514, "command"="set") -> ()  [unwired: 1 out]
                                }
                                frame 2 {
                                n1605 = Sort 1D Array(array=w4558) -> (sorted array=w4557:i32[])
                                n1606 = Reverse 1D Array(array=w4557) -> (reversed array=w4556:i32[])
                                n1607 = for {
                                tunnel: w4556 -> [w4562] mode=indexing
                                tunnel: [w4561] -> w4559
                                n1608 = call "waveformsDObuffer.vi"("command"="get") -> ("DO wf out"=w4564:digitalwaveform[])  [unwired: 1 in]
                                n1609 = Delete From Array(array=w4564, length=1, index=w4562) -> (deleted portion=w4561:digitalwaveform[], array with subset deleted=w4560:digitalwaveform[])
                                n1610 = call "waveformsDObuffer.vi"("DO wf in"=w4560, "command"="set") -> ()  [unwired: 1 out]
                                }
                                }
                                frame 3, Default {
                                }
                                frame 0 {
                                n1611 = call "2pparameters.vi"("command"="get") -> ("params out"=w4571:T12)  [unwired: 1 in]
                                n1612 = Unbundle By Name(w4571) -> ("autoshutter"=w4570:bool, "wavdet"=w4568:bool)
                                n1613 = case shown="True" w4570 {
                                tunnel: w4569 -> [_ w4575]
                                tunnel: w4568 -> [_ w4574]
                                tunnel: [_ w4573] -> w4567
                                frame False {
                                }
                                frame True {
                                n1614 = case shown="False" w4574 {
                                tunnel: w4575 -> [w4578 _]
                                tunnel: [w4577 _] -> w4573
                                frame False {
                                w4585 = u16 0 items=["unsigned binary", "offset binary", "2's complement"] ("data format (offset binary)")
                                n1615 = call "2pparameters.vi"("command"="get") -> ("params out"=w4592:T12)  [unwired: 1 in]
                                n1616 = call "waveformsDObuffer.vi"("command"="get") -> ("DO wf out"=w4579:digitalwaveform[])  [unwired: 1 in]
                                n1617 = Unbundle By Name(w4592) -> ("Pel"=w4594:sgl, "srate"=w4593:sgl)
                                n1618 = Initialize Array(sgl 1.0, w4594) -> (w4580:sgl[])
                                n1619 = Reciprocal(x=w4593) -> (1/x=w4587:sgl)
                                n1620 = Bundle By Name("Y"=w4580, "dt"=w4587) -> (w4583:waveform(sgl))  [unwired: 1 in]
                                n1621 = call-poly <vilib>:"Analog to Digital.vi"("data format (offset binary)"=w4585, "compress digital (T)"=TRUE, "full-scale range (pk-pk)"=1.0, "resolution (16 bit)"=1, "analog waveform"=w4583) -> ("digital waveform"=w4590:digitalwaveform)  [unwired: 3 in, 3 out]
                                n1622 = for {
                                tunnel: w4590 -> [w4599]
                                tunnel: w4578 -> [w4596] mode=indexing
                                tunnel: [w4595] -> w4577 mode=indexing
                                shift-right: [w4597] -> w4576
                                shift-left: w4579 -> [w4598]
                                n1623 = Index Array(array=w4598, index=w4596) -> (element=w4595:digitalwaveform)
                                n1624 = Replace Array Subset(array=w4598, new element=w4599, index=w4596) -> (w4597:digitalwaveform[])
                                }
                                n1625 = call "waveformsDObuffer.vi"("DO wf in"=w4576, "command"="set") -> ()  [unwired: 1 out]
                                }
                                frame True {
                                }
                                }
                                }
                                }
                                }
                                }
                                }
                                frame #8 {
                                n1626 = Build Array(w4603, w4602) -> (w4605:bool[])
                                n1627 = Boolean Array To Number(Boolean array=w4605) -> (number=w4604:u32)
                                n1628 = case shown="0" w4604 {
                                tunnel: w4601 -> [_ w4631 _ w4643]
                                tunnel: [_ w4630 _ w4641] -> w4600
                                frame 1 {
                                w4618 = 0.0 ("DOtab")
                                n1629 = call "2pparameters.vi"("command"="get") -> ("params out"=w4616:T12)  [unwired: 1 in]
                                n1630 = call "waveformparamsv2.vi"("command"="get") -> ("Params out"=w4626:T17)  [unwired: 4 in, 2 out]
                                n1631 = Unbundle By Name(w4626) -> ("DO parameters"=w4624:T20)
                                n1632 = Unbundle By Name(w4616) -> ("srate"=w4613:sgl, "Pel"=w4615:sgl)
                                n1633 = To Double Precision Float(number=w4613) -> (double precision float=w4611:dbl)
                                n1634 = To Double Precision Float(number=w4613) -> (double precision float=w4612:dbl)
                                n1635 = To Double Precision Float(number=w4615) -> (double precision float=w4607:dbl)
                                n1636 = Divide(x=w4612, y=w4607) -> (x/y=w4614:dbl)
                                n1637 = Index Array(array=w4624, index=0) -> (element=w4623:T21)
                                n1638 = Divide(x=1.0 ("Digital DC (%)"), y=w4607) -> (x/y=w4609:dbl)
                                n1639 = Multiply(x=100.0, y=w4609) -> (x*y=w4606:dbl)
                                n1640 = Bundle By Name(cluster=w4623, "Digital DC (%)"=w4606, "Digital phase"=w4618, "Digital Freq (Hz)"=w4614, "Sampling frequency (Hz)"=w4611, "Digital time offset (s)"=w4618, "padding value"=0.0, "matlab wave file"=path "LT", "DOtab"=0.0) -> (w4621:T21)
                                n1641 = Build Array(w4621) -> (w4620:T20)
                                n1642 = call "waveformparamsv2.vi"("command"="add DO", "add DO"=w4620) -> ()  [unwired: 3 in, 3 out]
                                }
                                frame 2 {
                                n1643 = call "waveformparamsv2.vi"("command"="get") -> ("Params out"=w4633:T17)  [unwired: 4 in, 2 out]
                                n1644 = in-place {
                                in-place-border: w4631 -> [w4637]
                                in-place-border: [w4636] -> w4630
                                n1645 = in-place-cluster #30(w4633) -> ("DO parameters"=w4639:T20)
                                n1646 = Delete From Array(array=w4639, length=1, index=w4637) -> (deleted portion=w4636:T20, array with subset deleted=w4638:T20)
                                n1647 = in-place-cluster #30("DO parameters"=w4638) -> (w4632:T17)
                                }
                                n1648 = call "waveformparamsv2.vi"("command"="set", "Params in"=w4632) -> ()  [unwired: 3 in, 3 out]
                                }
                                frame 3, Default {
                                }
                                frame 0 {
                                n1649 = local read "Measurement"() -> (w4645:T4)
                                n1650 = To Unsigned Long Integer(number=w4645) -> (unsigned 32bit integer=w4644:u32)
                                n1651 = case shown="5..7" w4644 {
                                tunnel: w4643 -> [_ w4647]
                                tunnel: [_ w4646] -> w4642
                                frame 0..4, Default {
                                }
                                frame 5..7 {
                                n1652 = stacked-sequence {
                                tunnel: w4647 -> [w4649 w4658]
                                tunnel: [w4648 _] -> w4646
                                frame #0 {
                                n1653 = call "waveformparamsv2.vi"("command"="get") -> ("Params out"=w4651:T17)  [unwired: 4 in, 2 out]
                                n1654 = Unbundle By Name(w4651) -> ("DO parameters"=w4652:T20)
                                n1655 = Index Array(array=w4652, index=w4649) -> (element=w4648:T21)
                                }
                                frame #1 {
                                w4666 = 0.0 ("padding value")
                                n1656 = call "2pparameters.vi"("command"="get") -> ("params out"=w4664:T12)  [unwired: 1 in]
                                n1657 = Unbundle By Name(w4664) -> ("srate"=w4662:sgl, "Pel"=w4663:sgl)
                                n1658 = To Double Precision Float(number=w4662) -> (double precision float=w4660:dbl)
                                n1659 = To Double Precision Float(number=w4662) -> (double precision float=w4661:dbl)
                                n1660 = To Double Precision Float(number=w4663) -> (double precision float=w4656:dbl)
                                n1661 = Divide(x=1.0 ("Digital DC (%)"), y=w4656) -> (x/y=w4655:dbl)
                                n1662 = Multiply(x=100.0, y=w4655) -> (x*y=w4654:dbl)
                                n1663 = Divide(x=w4661, y=w4656) -> (x/y=w4659:dbl)
                                n1664 = call "replace DO wf param.vi"("Digital Freq (Hz)"=w4659, "Digital DC (%)"=w4654, "Digital phase"=w4666, "Sampling frequency (Hz)"=w4660, "Digital time offset (s)"=w4666, "index of DO wave"=w4658, "padding value"=w4666, "matlab wave file"=path "LT" ("matlab wave number")) -> ()  [unwired: 3 in]
                                }
